vi "Custom Device CORE.vi"(8 "error in (no error)":errorcluster, 11 "CDW_MetaDataObj":refnum<class "NIVS_Consolidated_CDW_MetaDataObj.lvclass">) -> (0 "error out":errorcluster)   [LabVIEW 2015, in "NIVS_Consolidated_CDW_MetaDataObj.lvclass"]
doc: "This VI is the Core VI for the Custom Device Wizard.\n\nWritten by:\nStephan Daunke\n\nDate:\n2014/01/27\n\nCompany:\nNational Instruments Germany GmbH"
uses:
  NIVS_Consolidated_CDW_MetaDataObj.lvclass
  Action.ctl
  Internal data.ctl
  <resource>/dialog/NewProjectWizard/MetaDataObj/MetaDataObj.lvclass/MetaDataObj.ctl
  NIVS_Consolidated_CDW_MetaDataObj.lvclass/NIVS_Consolidated_CDW_MetaDataObj.ctl
  Template Classes/NIVS_CD Template/NIVS_CD Template.lvclass/NIVS_CD Template.ctl
  Utility folder.ctl
  CD Shared lvlib.ctl
  Common.ctl
  Add Item - Type.ctl
  CD System Explorer lvlib.ctl
  <vilib>/Utility/traverseref.llb/TRef TravTarget.ctl
  CD Engine lvlib.ctl
  Build Spec System Explorer.ctl
  Build Spec Engine.ctl
  <resource>/dialog/NewProjectWizard/MetaDataObj/Accessors/Read Project Root.vi
  Read CD Template.vi
  Template Classes/NIVS_CD Template/Read Extra Page Names.vi
  <resource>/dialog/NewProjectWizard/MetaDataObj/Accessors/Read Project Name.vi
  Utility folder.vi
  CD Shared lvlib.vi
  Common.vi
  CD System Explorer lvlib.vi
  CD Engine lvlib.vi
  <vilib>/Utility/config.llb/Write Key (String).vi
  <vilib>/Utility/config.llb/Write Key (Path).vi
  Build Spec System Explorer.vi
  Build Spec Engine.vi
  Template Classes/NIVS_CD Template/NIVS_CD Template.lvclass
  <vilib>/Utility/config.llb/NI_LVConfig.lvlib
  <vilib>/Utility/Data Type/NI_Data Type.lvlib
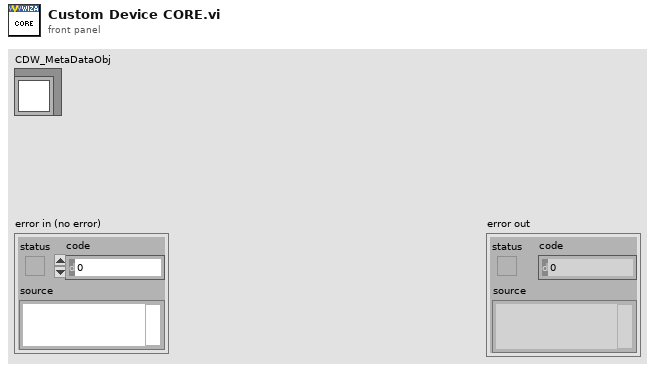
[diagram p1: front panel]
types:
  T1 = typedef "NIVS_Consolidated_CDW_MetaDataObj.lvclass/Internal data.ctl" = cluster{"CD GUID":string, "Extra Page GUIDs":string[], "System Explorer Library":refnum<vi>, "Shared Library":refnum<vi>, "Engine Library":refnum<vi>}
  T2 = typedef "NIVS_Consolidated_CDW_MetaDataObj.lvclass/Action.ctl" = enum16{"Project - Create Custom Device folder", "PC - Create GUID for each extra page", "PC-Utility - Create folder and copy -Copy .LLB to NI VeriStand dir-", "PC-Utility - Change -Copy .LLB to NI VeriStand dir-", "PC-Shared - Create folder and copy Constants.vi", "PC-Shared - Change Constants.vi content", "PC-Shared - Create library", "PC-Shared - Add folders and VIs to library", "PC-System Explorer - Create folder and copy templates", "PC-System Explorer - Create extra pages", "PC-System Explorer - Create library", "PC-System Explorer - Add folders and VIs to library", "PC-Engine - Create folder and copy the RT Template", "PC-Engine - Create library", "PC-Engine - Add virtual folders and VIs to library", "PC-XML - Create and change file", "PC-Help - Copy HTML Files", "Project - Read project file content", "Project - Edit Utility section", "Project - Edit XML section", "Project - Edit Engine Library section", "Project - Edit Shared Library section", "Project - Edit System Explorer Library section", "Project - Edit Custom Device Name", "Project - Edit System Explorer LLB Name", "Project - Edit Engine LLB OS dependent file name", "Project - Write new project file"}
  T3 = typedef "NIVS_Consolidated_CDW_MetaDataObj.lvclass/Utility folder.ctl" = enum16{"Utility.FolderName", "Utility.Copy .llb to NI VeriStand dir.FileName", "Utility.Copy .llb to NI VeriStand dir.FilePathAndName", "Utility.LLB Pre Build.FilePathAndName"}
  T4 = typedef "NIVS_Consolidated_CDW_MetaDataObj.lvclass/CD Shared lvlib.ctl" = enum16{"LibraryFileName", "LibraryFolderName", "ConstantsVI.VIPathAndName", "Shared.FolderName", "Shared.Types.FolderName", "Shared.Constants.VIName", "Shared.Constants.VITemplateName", "Shared.Constants.VITemplatePathAndName", "Shared.CompiledSettings.RelativePath", "Shared.Constants.RelativePath", "Shared.CompiledSettings.Name", "Shared.CompiledSettings.Name.NoExtension", "Shared.CompiledSettings.ClusterName"}
  T5 = typedef "NIVS_Consolidated_CDW_MetaDataObj.lvclass/Common.ctl" = enum16{"ProjectName", "TemplatesFolderName", "ProjectTemplatePathAndName", "TimingAndSyncFolderName", "CustomDeviceFolderName", "PathToTemplates"}
  T6 = typedef "NIVS_Consolidated_CDW_MetaDataObj.lvclass/Add Item - Type.ctl" = string
  T7 = typedef "NIVS_Consolidated_CDW_MetaDataObj.lvclass/CD System Explorer lvlib.ctl" = enum16{"LibraryFileName", "LibraryFolderName", "System Explorer.FolderName", "System Explorer.Dynamically Called.FolderName", "System Explorer.Dynamically Called.Extra Pages.FolderName", "System Explorer.Dynamically Called.Extra Pages.TemplatePathAndName", "System Explorer.Dynamically Called.Main Page.VIName", "System Explorer.Dynamically Called.Main Page.TemplatePathAndName", "System Explorer.Dynamically Called.Initialization VI.VIName", "System Explorer.Dynamically Called.Initialization VI.TemplatePathAndName", "System Explorer.SubVI.FolderName", "System Explorer.Types.FolderName", "System Explorer.ActionVIOnCompile.VIName", "System Explorer.ExportConfigRTM.VIName", "System Explorer.LoadHelpFile.VIName"}
  T8 = typedef "TRef TravTarget.ctl" = enum16{"FP", "BD", "Other"}
  T9 = typedef "NIVS_Consolidated_CDW_MetaDataObj.lvclass/CD Engine lvlib.ctl" = enum16{"LibraryFileName", "LibraryFolderName", "Engine.FolderName", "Engine.Init.FolderName", "Engine.Run.FolderName", "Engine.Shutdown.FolderName", "Types.FolderName", "Engine.RT Driver VI.TemplatePath", "Engine.RT Driver VI.FileName", "Engine.RTStateVariables.Name", "Engine.RTStateVariables.Name.NoExtension", "Engine.Async.NameExtension", "Engine.Async.TemplateName"}
  T10 = typedef "NIVS_Consolidated_CDW_MetaDataObj.lvclass/Build Spec System Explorer.ctl" = enum16{"Destinations.LLBFileName"}
  T11 = typedef "NIVS_Consolidated_CDW_MetaDataObj.lvclass/Build Spec Engine.ctl" = enum16{"Destinations.LLBWindowsFileName", "Destinations.LLBVxWorksFileName", "Destinations.LLBPharlapFileName", "Destinations.LLBLinuxARMFileName", "Destinations.LLBLinux64FileName"}
  T12 = enum16{"open", "replace", "create", "open or create", "replace or create", "replace or create with confirmation"}
  T13 = typedef "NI_LVConfig.lvlib/Config Data RefNum.ctl" = refnum<k1>
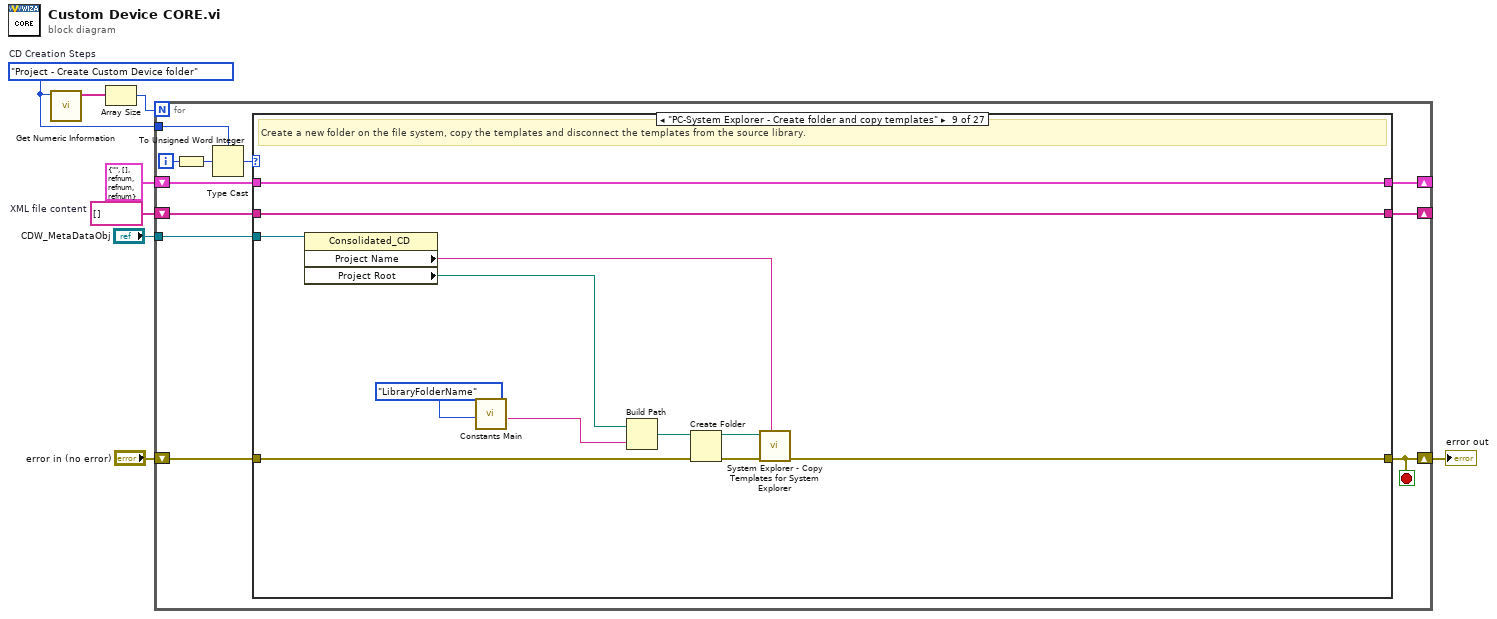
[diagram p0: block diagram]
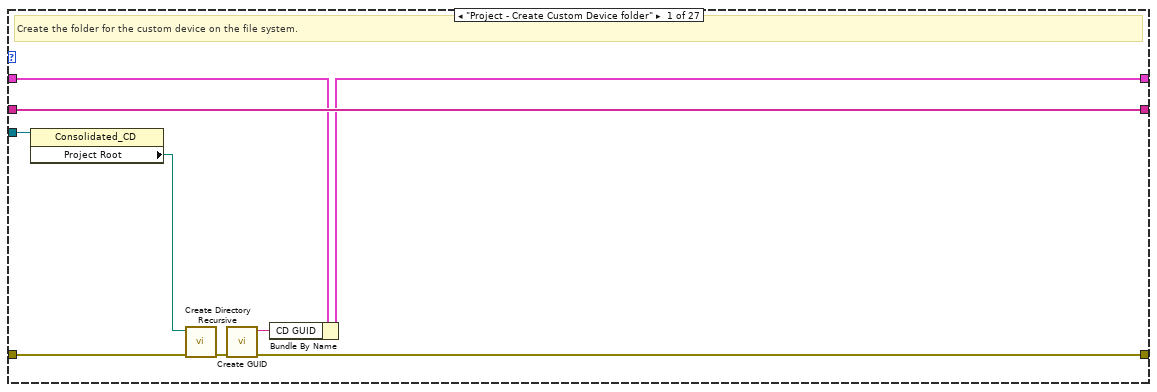
[diagram p2: hidden frame]
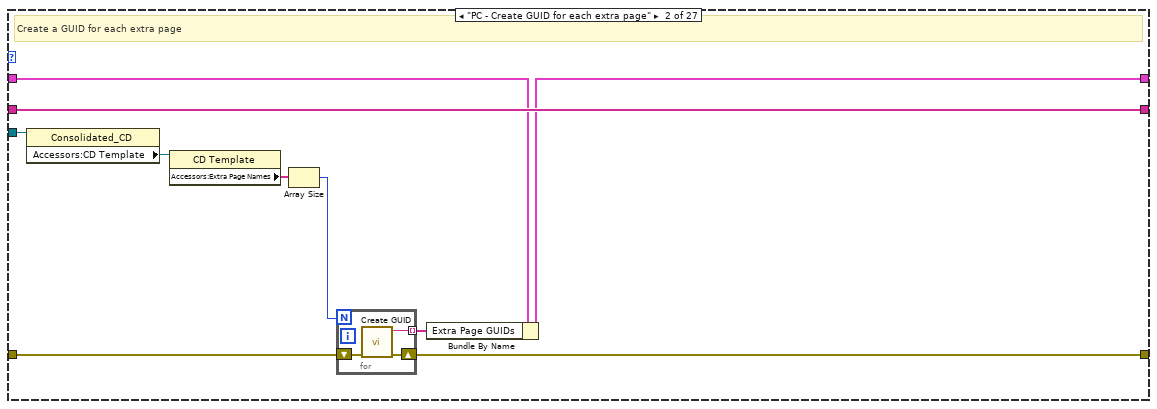
[diagram p3: hidden frame]
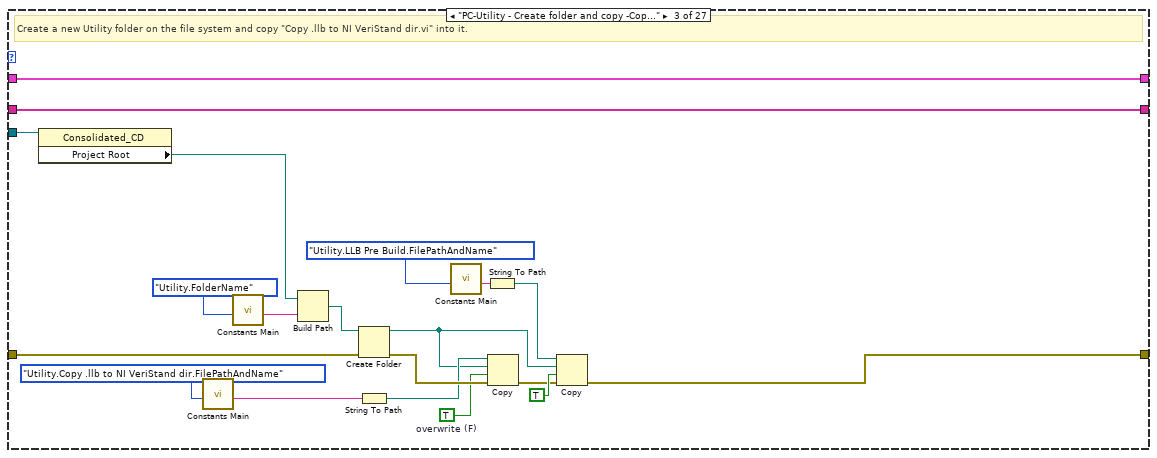
[diagram p4: hidden frame]
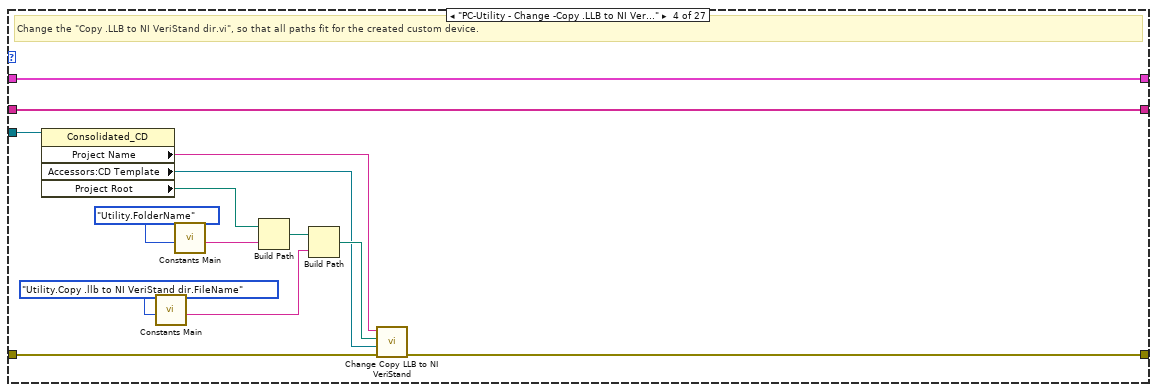
[diagram p5: hidden frame]
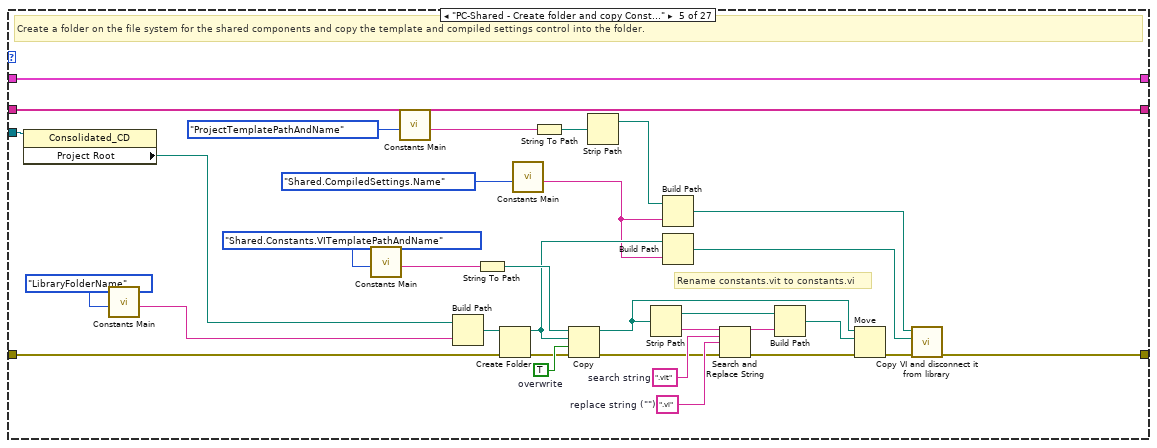
[diagram p6: hidden frame]
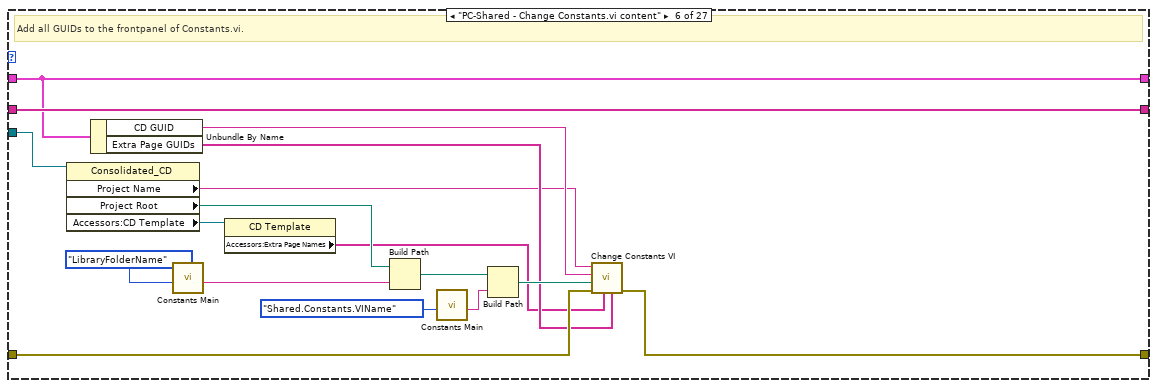
[diagram p7: hidden frame]
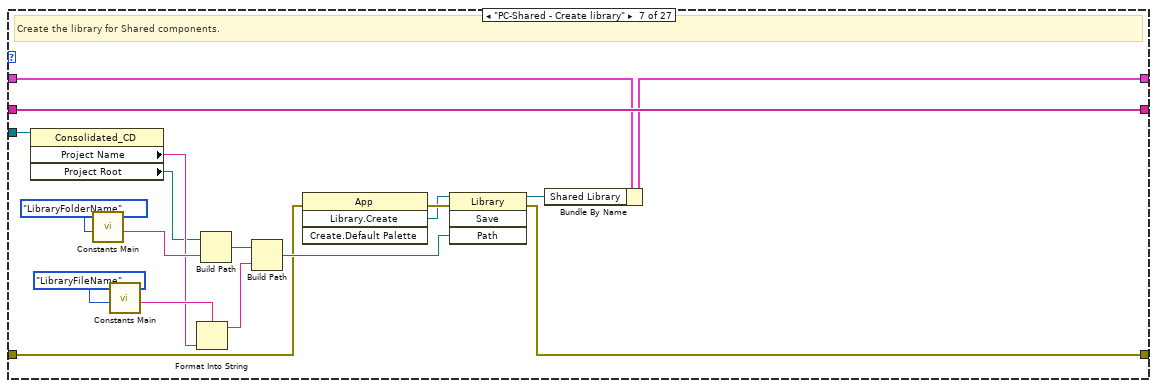
[diagram p8: hidden frame]
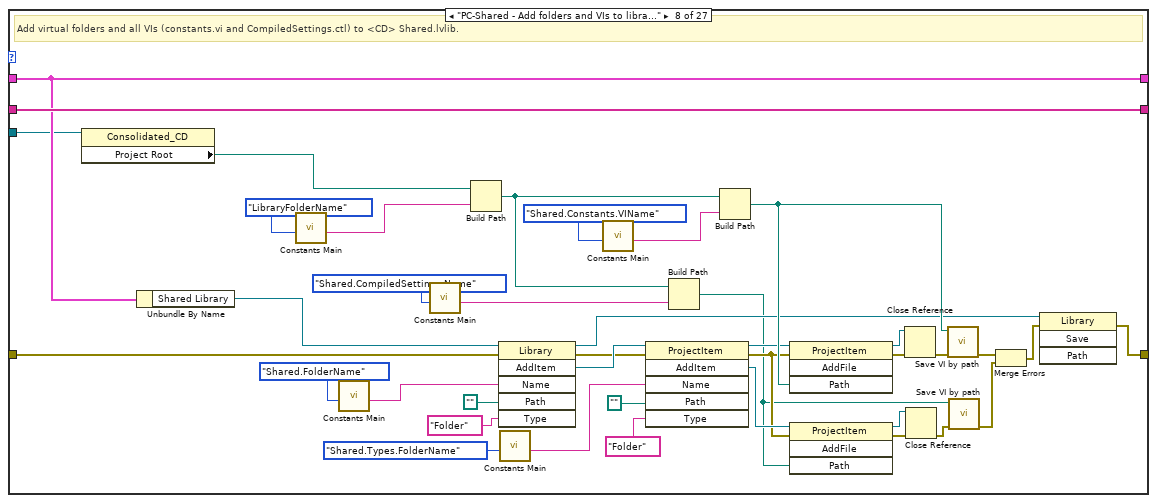
[diagram p9: hidden frame]
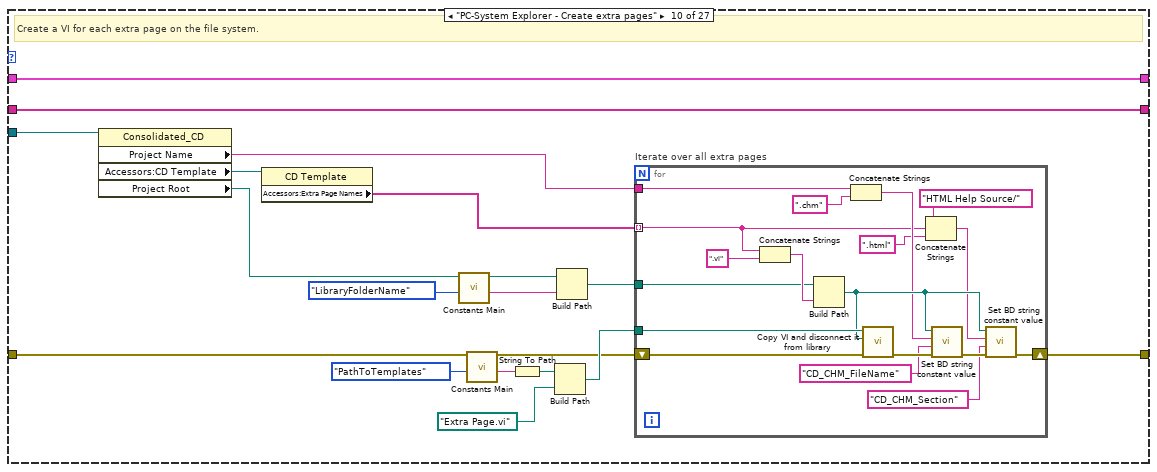
[diagram p10: hidden frame]
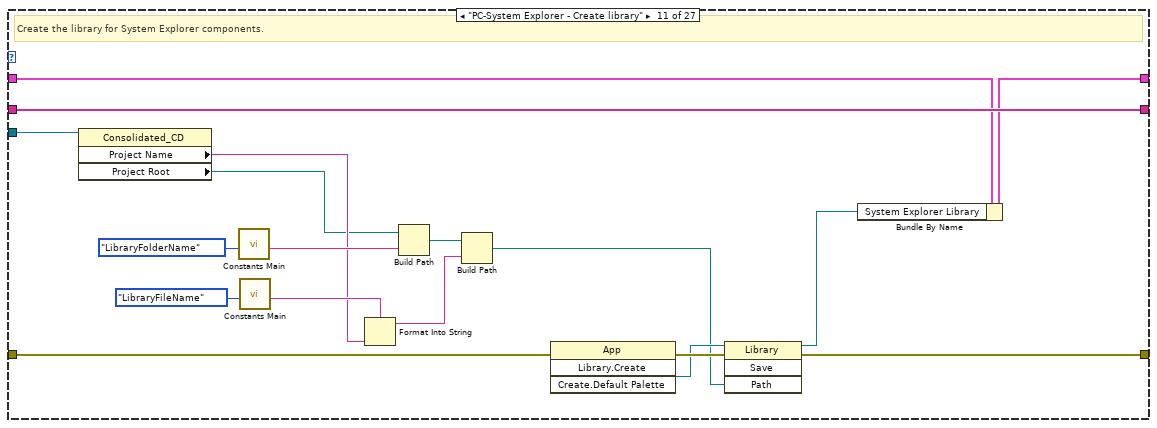
[diagram p11: hidden frame]
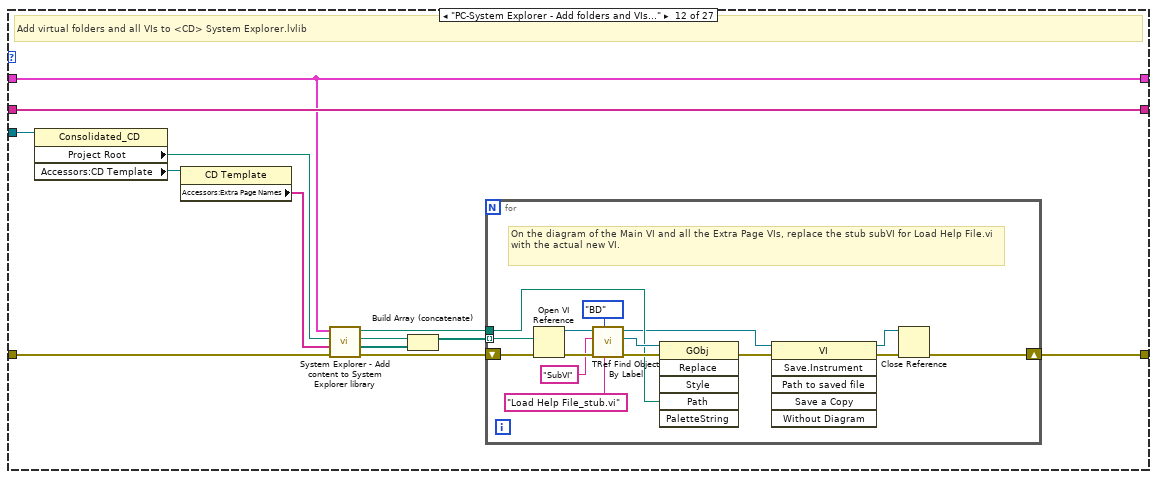
[diagram p12: hidden frame]
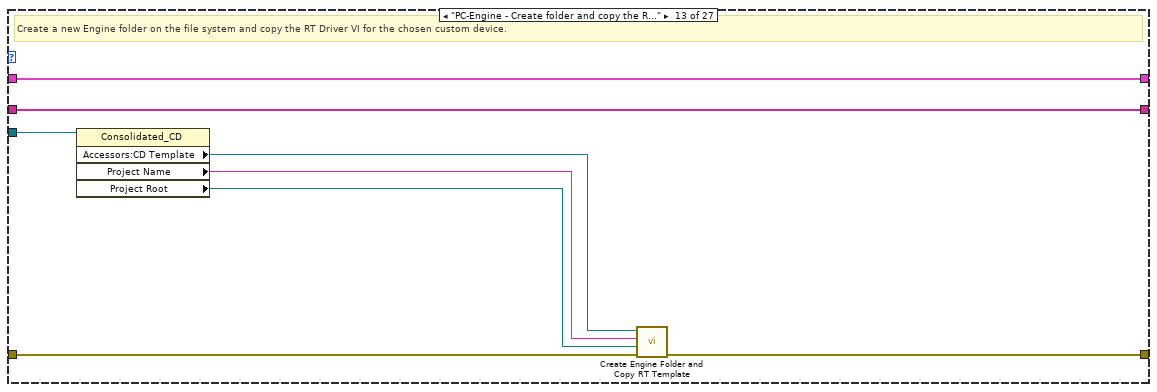
[diagram p13: hidden frame]
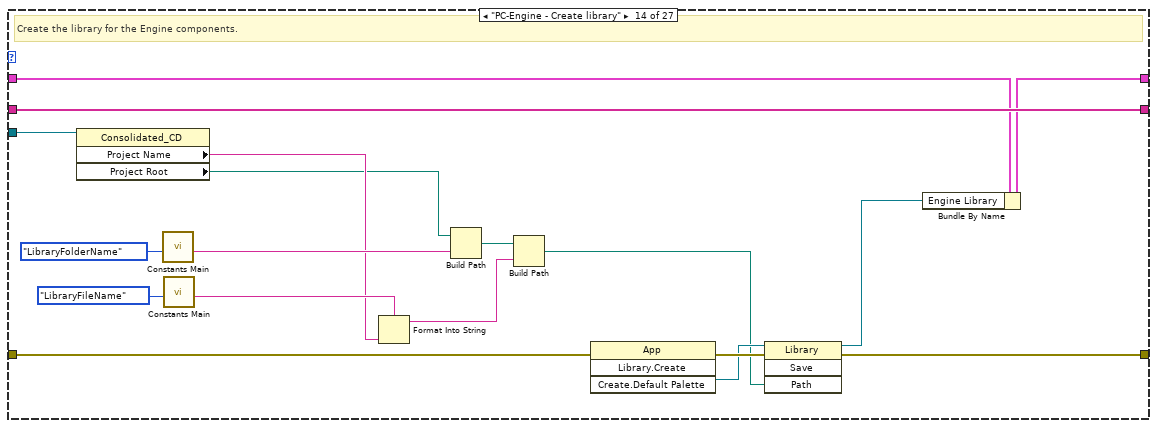
[diagram p14: hidden frame]
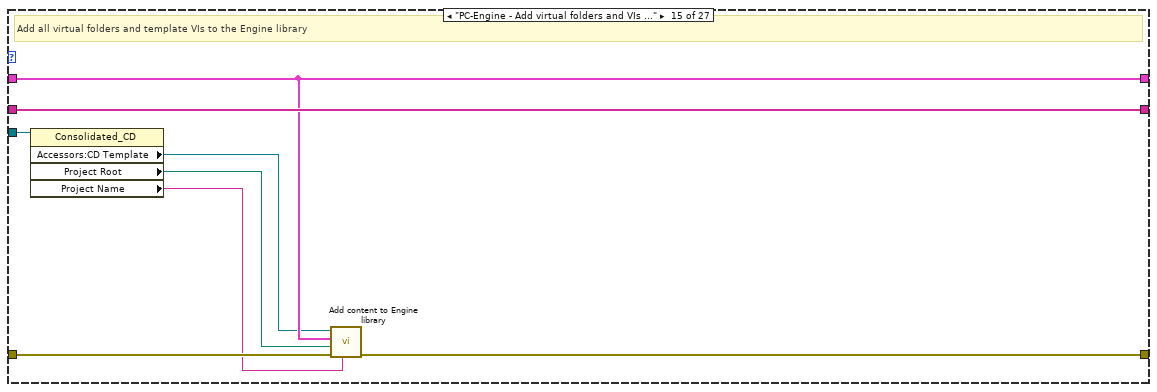
[diagram p15: hidden frame]
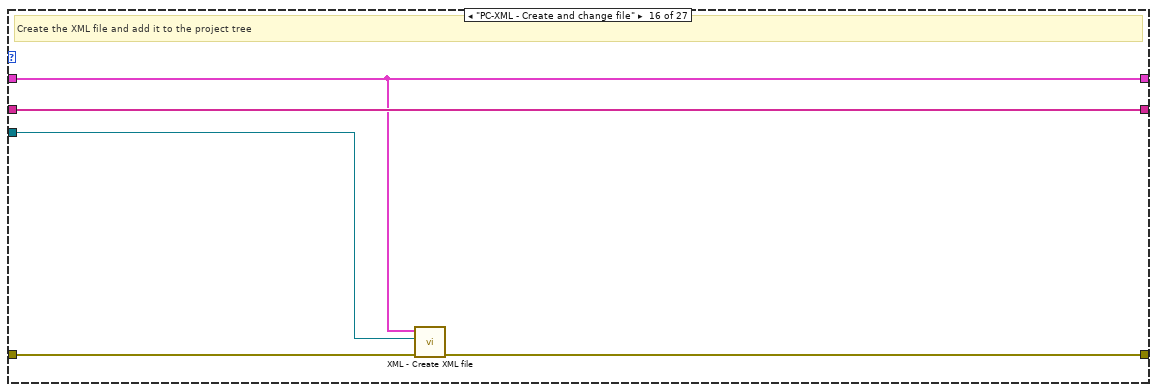
[diagram p16: hidden frame]
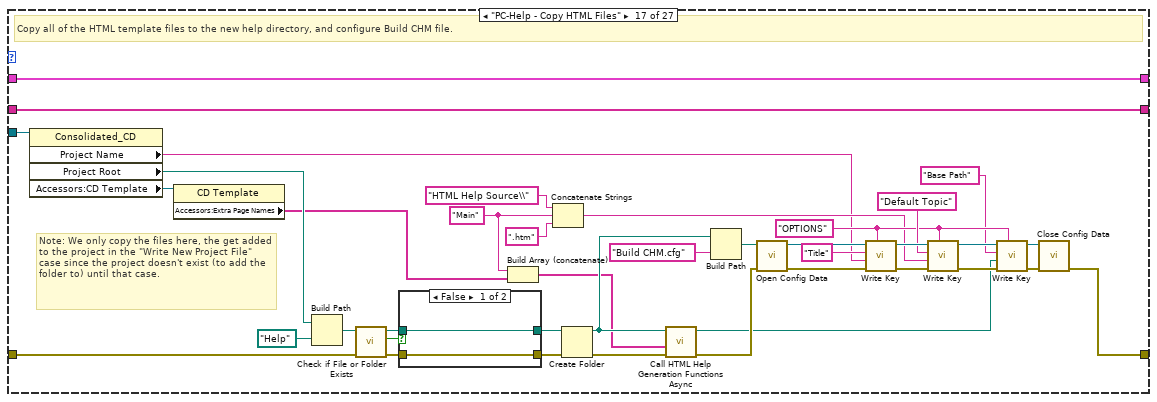
[diagram p17: hidden frame]
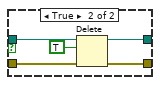
[diagram p18: hidden frame]
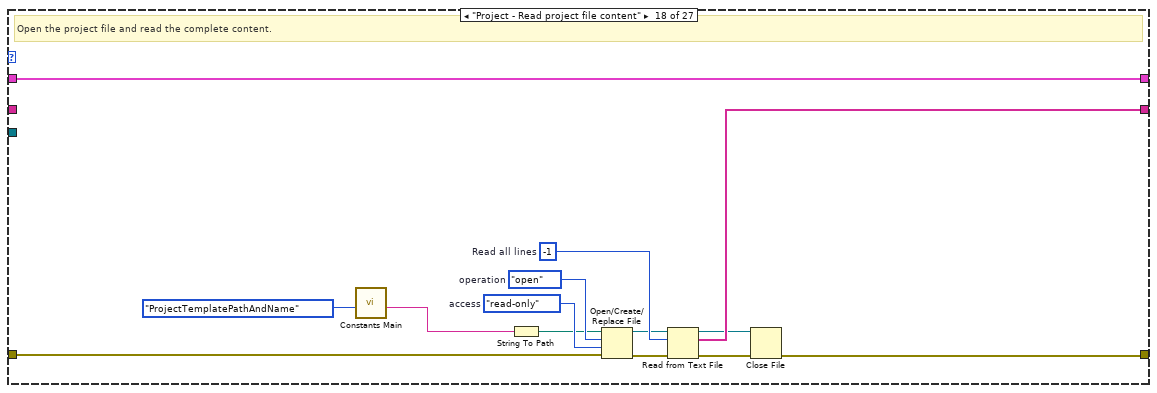
[diagram p19: hidden frame]
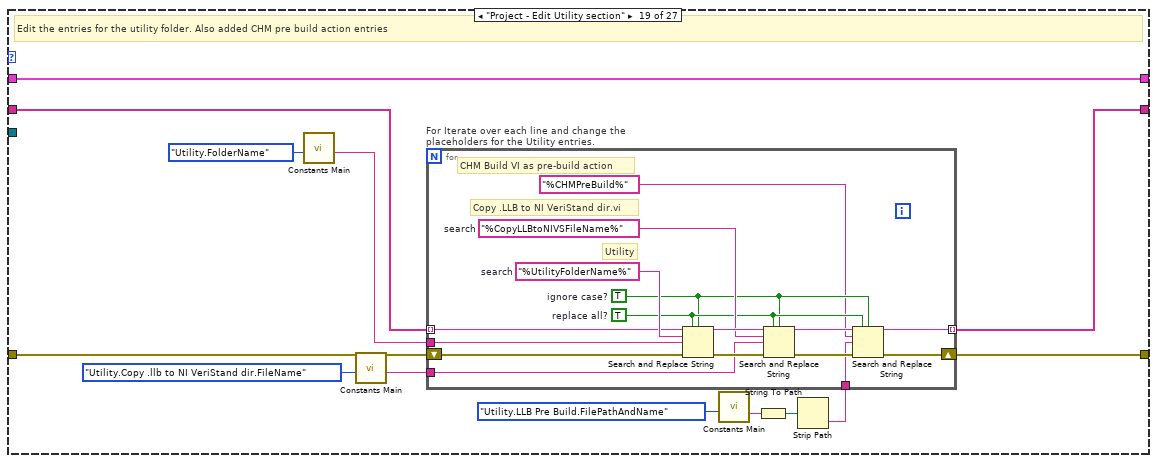
[diagram p20: hidden frame]
diagram:
  w4 = Action."Project - Create Custom Device folder"  # CD Creation Steps
  w5 = string[] []  # XML file content
  n1 = call <vilib>:"Get Numeric Information.vi"("Variant"=w4) -> ("Enum Names"=w3:string[])  [unwired: 7 in, 3 out]
  n2 = Array Size(array=w3) -> (size(s)=w2:i32)
  n3 = for {
    N: w2 -> [_]
    shift-right: [w16] -> _
    shift-left: T1 {"CD GUID"="", "Extra Page GUIDs"=[], "System Explorer Library"=refnum, "Shared Library"=refnum, "Engine Library"=refnum} ("CD Wizard - Internal Data") -> [w18]
    shift-right: [w15] -> _
    shift-left: w5 -> [w17]
    shift-right: [w14] -> w6
    shift-left: "error in (no error)" -> [w19]
    tunnel: w4 -> [w12]
    tunnel: "CDW_MetaDataObj" -> [w11]
    i -> [w13]
    stop <- w14 stop-if-true
    n4 = To Unsigned Word Integer(number=w13) -> (unsigned 16bit integer=w9:u16)
    n5 = Type Cast(type=w12, x=w9) -> (*(type *) &x=w10:T2)
    n6 = case shown="\"PC-System Explorer - Create folder and copy templates\"" w10 {
      tunnel: w19 -> [w24 w37 w43 w63 w78 w118 w129 w145 w183 w200 w233 w259 w282 w287 w308 w313 w331 w361 w374 w406 w425 w429 w459 w493 w504 w522 w560]
      tunnel: [w25 w36 w47 w69 w80 w124 w130 w163 w188 w210 w234 w254 w281 w290 w307 w312 w330 w367 w383 w411 w424 w439 w463 w492 w511 w534 w567] -> w14
      tunnel: w18 -> [w22 w34 w46 w67 w79 w115 w133 w164 w187 w209 w239 w257 w280 w294 w305 w311 w326 w373 w386 w408 w423 w430 w460 w489 w508 w540 w592]
      tunnel: w17 -> [w28 w38 w61 w75 w108 w125 w143 w182 w194 w211 w247 w260 w283 w301 w309 w314 w353 _ w385 w410 w422 w434 w461 w490 w506 w535 w586]
      tunnel: [w27 w33 w46 w67 w79 w115 w132 w164 w187 w209 w240 w257 w280 w293 w305 w311 w326 w373 w386 w408 w423 w430 w460 w489 w508 w540 w592] -> w16
      tunnel: [w28 w38 w61 w75 w108 w125 w143 w182 w194 w211 w247 w260 w283 w301 w309 w314 w353 w366 w384 w409 w426 w440 w462 w491 w505 w523 w586] -> w15
      tunnel: w11 -> [w21 w32 w45 w66 w77 w117 w128 w147 w186 w199 w232 w253 w279 w286 w306 w310 w319 _ _ w405 w421 w428 w458 w488 w503 w521 w559]
      frame "Project - Create Custom Device folder" {
        # "Create the folder for the custom device on the file system."
        n7 = property class="Consolidated_CD"(reference=w21) -> ("Project Root"=w20:path)  [unwired: 1 in, 2 out]
        n8 = call <vilib>:"Create Directory Recursive.vi"("error in (no error)"=w24, "directory"=w20) -> ("error out"=w23:errorcluster)  [unwired: 3 in, 2 out]
        n9 = call "Create GUID.vi"("error in (no error)"=w23) -> ("error out"=w25:errorcluster, "Generated GUID"=w26:string)  [unwired: 9 in]
        n10 = Bundle By Name(cluster=w22, "CD GUID"=w26) -> (w27:T1)
      }
      frame "PC - Create GUID for each extra page" {
        # "Create a GUID for each extra page"
        n11 = property class="Consolidated_CD"(reference=w32) -> ("Accessors:CD Template"=w31:refnum<class "NIVS_CD Template.lvclass">)  [unwired: 1 in, 2 out]
        n12 = property class="CD Template"(reference=w31) -> ("Accessors:Extra Page Names"=w30:string[])  [unwired: 1 in, 2 out]
        n13 = Array Size(array=w30) -> (size(s)=w29:i32)
        n14 = for {
          N: w29 -> [_]
          shift-right: [w40] -> w36
          shift-left: w37 -> [w41]
          tunnel: [w39] -> w35 mode=indexing
          n15 = call "Create GUID.vi"("error in (no error)"=w41) -> ("error out"=w40:errorcluster, "Generated GUID"=w39:string)  [unwired: 9 in]
        }
        n16 = Bundle By Name(cluster=w34, "Extra Page GUIDs"=w35) -> (w33:T1)
      }
      frame "PC-Utility - Create folder and copy -Copy .LLB to NI VeriStand dir-" {
        w58 = TRUE  # overwrite (F)
        # "Create a new Utility folder on the file system and copy \"Copy .llb to NI VeriStand dir.vi\" into it."
        n17 = property class="Consolidated_CD"(reference=w45) -> ("Project Root"=w44:path)  [unwired: 1 in, 2 out]
        n18 = call-poly "Constants Main.vi"("Action"=Utility_folder."Utility.Copy .llb to NI VeriStand dir.FilePathAndName") -> ("Output"=w56:string)  [unwired: 10 in]
        n19 = call-poly "Constants Main.vi"("Action"=Utility_folder."Utility.FolderName") -> ("Output"=w53:string)  [unwired: 10 in]
        n20 = Build Path(base path=w44, name or relative path=w53) -> (appended path=w60:path)
        n21 = Create Folder(path (use dialog)=w60, error in=w43) -> (created path=w52:path, error out=w59:errorcluster)  [unwired: 1 in, 1 out]
        n22 = String To Path(string=w56) -> (path=w55:path)
        n23 = call-poly "Constants Main.vi"("Action"=Utility_folder."Utility.LLB Pre Build.FilePathAndName") -> ("Output"=w50:string)  [unwired: 10 in]
        n24 = String To Path(string=w50) -> (path=w49:path)
        n25 = Copy(8:w59, 9:w58, 10:w52, 11:w55) -> (0:w42:errorcluster)  [unwired: 3 out]
        n26 = Copy(8:w42, 9:TRUE ("overwrite (F)"), 10:w52, 11:w49) -> (0:w47:errorcluster)  [unwired: 3 out]
      }
      frame "PC-Utility - Change -Copy .LLB to NI VeriStand dir-" {
        # "Change the \"Copy .LLB to NI VeriStand dir.vi\", so that all paths fit for the created custom device."
        n27 = property class="Consolidated_CD"(reference=w66) -> ("Project Name"=w65:string, "Accessors:CD Template"=w64:refnum<class "NIVS_CD Template.lvclass">, "Project Root"=w62:path)  [unwired: 1 in, 2 out]
        n28 = call-poly "Constants Main.vi"("Action"=Utility_folder."Utility.Copy .llb to NI VeriStand dir.FileName") -> ("Output"=w70:string)  [unwired: 10 in]
        n29 = call-poly "Constants Main.vi"("Action"=Utility_folder."Utility.FolderName") -> ("Output"=w72:string)  [unwired: 10 in]
        n30 = Build Path(base path=w62, name or relative path=w72) -> (appended path=w71:path)
        n31 = Build Path(base path=w71, name or relative path=w70) -> (appended path=w68:path)
        n32 = call "Change Copy LLB to NI VeriStand.vi"("error in (no error)"=w63, "CD Template"=w64, "Copy .LLB to ... path"=w68, "CD Name"=w65) -> ("error out"=w69:errorcluster)  [unwired: 7 in]
      }
      frame "PC-Shared - Create folder and copy Constants.vi" {
        w97 = ".vi"  # replace string ("")
        w98 = ".vit"  # search string
        w102 = TRUE  # overwrite
        # "Rename constants.vit to constants.vi"
        # "Create a folder on the file system for the shared components and copy the template and compiled settings control into the folder."
        n33 = property class="Consolidated_CD"(reference=w77) -> ("Project Root"=w76:path)  [unwired: 1 in, 2 out]
        n34 = call-poly "Constants Main.vi"("Action"=CD_Shared_lvlib."LibraryFolderName") -> ("Output"=w105:string)  [unwired: 10 in]
        n35 = call-poly "Constants Main.vi"("Action"=CD_Shared_lvlib."Shared.Constants.VITemplatePathAndName") -> ("Output"=w103:string)  [unwired: 10 in]
        n36 = call-poly "Constants Main.vi"("Action"=Common."ProjectTemplatePathAndName") -> ("Output"=w89:string)  [unwired: 10 in]
        n37 = Build Path(base path=w76, name or relative path=w105) -> (appended path=w107:path)
        n38 = String To Path(string=w103) -> (path=w95:path)
        n39 = Create Folder(path (use dialog)=w107, error in=w78) -> (created path=w86:path, error out=w96:errorcluster)  [unwired: 1 in, 1 out]
        n40 = call-poly "Constants Main.vi"("Action"=CD_Shared_lvlib."Shared.CompiledSettings.Name") -> ("Output"=w81:string)  [unwired: 10 in]
        n41 = String To Path(string=w89) -> (path=w88:path)
        n42 = Copy(8:w96, 9:w102, 10:w86, 11:w95) -> (0:w94:errorcluster, 3:w91:path)  [unwired: 2 out]
        n43 = Strip Path(path=w88) -> (stripped path=w87:path)  [unwired: 1 out]
        n44 = Strip Path(path=w91) -> (stripped path=w101:path, name=w100:string)
        n45 = Build Path(base path=w87, name or relative path=w81) -> (appended path=w85:path)
        n46 = Build Path(base path=w86, name or relative path=w81) -> (appended path=w84:path)
        n47 = Search and Replace String(input string=w100, search string=w98, replace string=w97, error in=w94) -> (result string=w99:string, error out=w93:errorcluster)  [unwired: 4 in, 2 out]
        n48 = Build Path(base path=w101, name or relative path=w99) -> (appended path=w92:path)
        n49 = Move(source path=w91, error in=w93, 10:w92) -> (error out=w83:errorcluster)  [unwired: 2 in, 2 out]
        n50 = call "Copy VI and disconnect it from library.vi"("error in (no error)"=w83, "VI Target Path"=w84, "VI Source Path"=w85) -> ("error out"=w80:errorcluster)  [unwired: 8 in]
      }
      frame "PC-Shared - Change Constants.vi content" {
        # "Add all GUIDs to the frontpanel of Constants.vi."
        n51 = property class="Consolidated_CD"(reference=w117) -> ("Project Name"=w111:string, "Project Root"=w116:path, "Accessors:CD Template"=w110:refnum<class "NIVS_CD Template.lvclass">)  [unwired: 1 in, 2 out]
        n52 = Unbundle By Name(w115) -> ("CD GUID"=w113:string, "Extra Page GUIDs"=w112:string[])
        n53 = call-poly "Constants Main.vi"("Action"=CD_Shared_lvlib."LibraryFolderName") -> ("Output"=w119:string)  [unwired: 10 in]
        n54 = property class="CD Template"(reference=w110) -> ("Accessors:Extra Page Names"=w109:string[])  [unwired: 1 in, 2 out]
        n55 = Build Path(base path=w116, name or relative path=w119) -> (appended path=w123:path)
        n56 = call-poly "Constants Main.vi"("Action"=CD_Shared_lvlib."Shared.Constants.VIName") -> ("Output"=w121:string)  [unwired: 10 in]
        n57 = Build Path(base path=w123, name or relative path=w121) -> (appended path=w114:path)
        n58 = call "Change Constants VI.vi"("Extra Page GUIDs"=w112, "Extra Page Names"=w109, "error in (no error)"=w118, "Constants.vi path"=w114, "CD GUID"=w113, "CD Name"=w111) -> ("error out"=w124:errorcluster)  [unwired: 5 in]
      }
      frame "PC-Shared - Create library" {
        # "Create the library for Shared components."
        n59 = property class="Consolidated_CD"(reference=w128) -> ("Project Name"=w127:string, "Project Root"=w126:path)  [unwired: 1 in, 2 out]
        n60 = call-poly "Constants Main.vi"("Action"=CD_Shared_lvlib."LibraryFolderName") -> ("Output"=w137:string)  [unwired: 10 in]
        n61 = call-poly "Constants Main.vi"("Action"=CD_Shared_lvlib."LibraryFileName") -> ("Output"=w138:string)  [unwired: 10 in]
        n62 = Format Into String(format string=w138, w127) -> (resulting string=w141:string)  [unwired: 2 in, 1 out]
        n63 = Build Path(base path=w126, name or relative path=w137) -> (appended path=w142:path)
        n64 = Build Path(base path=w142, name or relative path=w141) -> (appended path=w134:path)
        n65 = invoke class="App" method="Library.Create"(error in=w129) -> (error out=w136:errorcluster, "Create Library"=w135:refnum<vi>)  [unwired: 3 in, 2 out]
        n66 = invoke class="Library" method="Save"(reference=w135, error in=w136, "Path"=w134) -> (reference out=w131:refnum<vi>, error out=w130:errorcluster)  [unwired: 1 in, 2 out]
        n67 = Bundle By Name(cluster=w133, "Shared Library"=w131) -> (w132:T1)
      }
      frame "PC-Shared - Add folders and VIs to library" {
        # "Add virtual folders and all VIs (constants.vi and CompiledSettings.ctl) to <CD> Shared.lvlib."
        n68 = property class="Consolidated_CD"(reference=w147) -> ("Project Root"=w146:path)  [unwired: 1 in, 2 out]
        n69 = Unbundle By Name(w164) -> ("Shared Library"=w166:refnum<vi>)
        n70 = call-poly "Constants Main.vi"("Action"=CD_Shared_lvlib."LibraryFolderName") -> ("Output"=w160:string)  [unwired: 10 in]
        n71 = call-poly "Constants Main.vi"("Action"=CD_Shared_lvlib."Shared.FolderName") -> ("Output"=w161:string)  [unwired: 10 in]
        n72 = call-poly "Constants Main.vi"("Action"=CD_Shared_lvlib."Shared.CompiledSettings.Name") -> ("Output"=w152:string)  [unwired: 10 in]
        n73 = Build Path(base path=w146, name or relative path=w160) -> (appended path=w157:path)
        n74 = invoke class="Library" method="AddItem"(reference=w166, error in=w145, "Name"=w161, "Path"=path "", "Type"=T6 "Folder" ("Add Item - Type")) -> (reference out=w172:refnum<vi>, error out=w167:errorcluster, "AddItem"=w169:refnum<vi>)  [unwired: 1 in, 3 out]
        n75 = call-poly "Constants Main.vi"("Action"=CD_Shared_lvlib."Shared.Types.FolderName") -> ("Output"=w180:string)  [unwired: 10 in]
        n76 = call-poly "Constants Main.vi"("Action"=CD_Shared_lvlib."Shared.Constants.VIName") -> ("Output"=w148:string)  [unwired: 10 in]
        n77 = invoke class="ProjectItem" method="AddItem"(reference=w169, error in=w167, "Name"=w180, "Path"=path "", "Type"=T6 "Folder" ("Add Item - Type")) -> (reference out=w171:refnum<vi>, error out=w158:errorcluster, "AddItem"=w159:refnum<vi>)  [unwired: 1 in, 3 out]
        n78 = Build Path(base path=w157, name or relative path=w152) -> (appended path=w156:path)
        n79 = Build Path(base path=w157, name or relative path=w148) -> (appended path=w173:path)
        n80 = invoke class="ProjectItem" method="AddFile"(reference=w171, error in=w158, "Path"=w173) -> (reference out=w176:refnum<vi>, error out=w175:errorcluster)  [unwired: 1 in, 2 out]
        n81 = invoke class="ProjectItem" method="AddFile"(reference=w159, error in=w158, "Path"=w156) -> (reference out=w150:refnum<vi>, error out=w149:errorcluster)  [unwired: 1 in, 2 out]
        n82 = Close Reference(reference=w176, error in (no error)=w175) -> (error out=w177:errorcluster)
        n83 = Close Reference(reference=w150, error in (no error)=w149) -> (error out=w151:errorcluster)
        n84 = call "Save VI by path.vi"("error in (no error)"=w177, "VI path"=w173) -> ("error out"=w174:errorcluster)  [unwired: 9 in]
        n85 = call "Save VI by path.vi"("error in (no error)"=w151, "VI path"=w156) -> ("error out"=w154:errorcluster)  [unwired: 9 in]
        n86 = Merge Errors(w174, w154) -> (w155:errorcluster)
        n87 = invoke class="Library" method="Save"(reference=w172, error in=w155) -> (error out=w163:errorcluster)  [unwired: 2 in, 3 out]
      }
      frame "PC-System Explorer - Create folder and copy templates" {
        # "Create a new folder on the file system, copy the templates and disconnect the templates from the source library."
        n88 = property class="Consolidated_CD"(reference=w186) -> ("Project Name"=w185:string, "Project Root"=w184:path)  [unwired: 1 in, 2 out]
        n89 = call-poly "Constants Main.vi"("Action"=CD_System_Explorer_lvlib."LibraryFolderName") -> ("Output"=w191:string)  [unwired: 10 in]
        n90 = Build Path(base path=w184, name or relative path=w191) -> (appended path=w193:path)
        n91 = Create Folder(path (use dialog)=w193, error in=w183) -> (created path=w189:path, error out=w190:errorcluster)  [unwired: 1 in, 1 out]
        n92 = call "System Explorer - Copy Templates for System Explorer.vi"("CD Name"=w185, "error in (no error)"=w190, "System Explorer folder"=w189) -> ("error out"=w188:errorcluster)  [unwired: 8 in]
      }
      frame "PC-System Explorer - Create extra pages" {
        # "Create a VI for each extra page on the file system."
        n93 = property class="Consolidated_CD"(reference=w199) -> ("Project Name"=w198:string, "Accessors:CD Template"=w197:refnum<class "NIVS_CD Template.lvclass">, "Project Root"=w195:path)  [unwired: 1 in, 2 out]
        n94 = property class="CD Template"(reference=w197) -> ("Accessors:Extra Page Names"=w196:string[])  [unwired: 1 in, 2 out]
        n95 = call-poly "Constants Main.vi"("Action"=CD_System_Explorer_lvlib."LibraryFolderName") -> ("Output"=w207:string)  [unwired: 10 in]
        n96 = call-poly "Constants Main.vi"("Action"=Common."PathToTemplates") -> ("Output"=w203:string)  [unwired: 10 in]
        n97 = String To Path(string=w203) -> (path=w202:path)
        n98 = Build Path(base path=w202, name or relative path=path "Extra Page.vi") -> (appended path=w208:path)
        n99 = Build Path(base path=w195, name or relative path=w207) -> (appended path=w205:path)
        n100 = for "Iterate over all extra pages" {
          tunnel: w196 -> [w213] mode=indexing
          shift-right: [w218] -> w210
          shift-left: w200 -> [w227]
          tunnel: w205 -> [w225]
          tunnel: w208 -> [w226]
          tunnel: w198 -> [w222]
          n101 = Concatenate Strings(w213, ".vi") -> (w228:string)
          n102 = Build Path(base path=w225, name or relative path=w228) -> (appended path=w220:path)
          n103 = Concatenate Strings(w222, ".chm" ("string")) -> (w217:string)
          n104 = call "Copy VI and disconnect it from library.vi"("error in (no error)"=w227, "VI Target Path"=w220, "VI Source Path"=w226) -> ("error out"=w224:errorcluster)  [unwired: 8 in]
          n105 = Concatenate Strings("HTML Help Source/" ("string"), w213, ".html" ("string")) -> (w215:string)
          n106 = call "Set BD string constant value.vi"("error in (no error)"=w224, "Name of string constant"="CD_CHM_FileName", "New String Value"=w217, "Path to VI"=w220) -> ("error out"=w221:errorcluster)  [unwired: 7 in]
          n107 = call "Set BD string constant value.vi"("error in (no error)"=w221, "Name of string constant"="CD_CHM_Section", "New String Value"=w215, "Path to VI"=w220) -> ("error out"=w218:errorcluster)  [unwired: 7 in]
        }
      }
      frame "PC-System Explorer - Create library" {
        # "Create the library for System Explorer components."
        n108 = property class="Consolidated_CD"(reference=w232) -> ("Project Name"=w231:string, "Project Root"=w230:path)  [unwired: 1 in, 2 out]
        n109 = call-poly "Constants Main.vi"("Action"=CD_System_Explorer_lvlib."LibraryFolderName") -> ("Output"=w243:string)  [unwired: 10 in]
        n110 = call-poly "Constants Main.vi"("Action"=CD_System_Explorer_lvlib."LibraryFileName") -> ("Output"=w244:string)  [unwired: 10 in]
        n111 = Format Into String(format string=w244, w231) -> (resulting string=w245:string)  [unwired: 2 in, 1 out]
        n112 = Build Path(base path=w230, name or relative path=w243) -> (appended path=w246:path)
        n113 = Build Path(base path=w246, name or relative path=w245) -> (appended path=w235:path)
        n114 = invoke class="App" method="Library.Create"(error in=w233) -> (error out=w238:errorcluster, "Create Library"=w237:refnum<vi>)  [unwired: 3 in, 2 out]
        n115 = invoke class="Library" method="Save"(reference=w237, error in=w238, "Path"=w235) -> (reference out=w236:refnum<vi>, error out=w234:errorcluster)  [unwired: 1 in, 2 out]
        n116 = Bundle By Name(cluster=w239, "System Explorer Library"=w236) -> (w240:T1)
      }
      frame "PC-System Explorer - Add folders and VIs to library" {
        # "Add virtual folders and all VIs to <CD> System Explorer.lvlib"
        n117 = property class="Consolidated_CD"(reference=w253) -> ("Project Root"=w252:path, "Accessors:CD Template"=w251:refnum<class "NIVS_CD Template.lvclass">)  [unwired: 1 in, 2 out]
        n118 = property class="CD Template"(reference=w251) -> ("Accessors:Extra Page Names"=w250:string[])  [unwired: 1 in, 2 out]
        n119 = call "System Explorer - Add content to System Explorer library.vi"("error in (no error)"=w259, "Extra Page Names"=w250, "Project Root"=w252, "CD Wizard - Internal Data"=w257) -> ("error out"=w258:errorcluster, "Extra Page VIs"=w248:path[], "System Explorer Main VI"=w256:path, "Load Help File VI"=w255:path)  [unwired: 4 in]
        n120 = Build Array (concatenate)(w256, w248) -> (w249:path[])
        n121 = for {
          tunnel: w249 -> [w266] mode=indexing
          tunnel: w255 -> [w265]
          shift-right: [w262] -> w254
          shift-left: w258 -> [w275]
          # "On the diagram of the Main VI and all the Extra Page VIs, replace the stub subVI for Load Help File.vi with the actual new VI."
          n122 = Open VI Reference(vi path=w266, error in (no error)=w275) -> (vi reference=w272:refnum<vi>, error out=w274:errorcluster)  [unwired: 4 in]
          n123 = call <vilib>:"TRef Find Object By Label.vi"("Label"="Load Help File_stub.vi", "Traverse Target"=TRef_TravTarget."BD", "error in (no error)"=w274, "Class Name"="SubVI", "VI Ref"=w272) -> ("error out"=w273:errorcluster, "Found Obj Ref"=w267:refnum<vi>, "dup VI Ref"=w263:refnum<vi>)  [unwired: 3 in, 1 out]
          n124 = invoke class="GObj" method="Replace"(reference=w267, error in=w273, "Path"=w265) -> (error out=w268:errorcluster)  [unwired: 3 in, 5 out]
          n125 = invoke class="VI" method="Save.Instrument"(reference=w263, error in=w268) -> (reference out=w261:refnum<vi>, error out=w264:errorcluster)  [unwired: 4 in, 4 out]
          n126 = Close Reference(reference=w261, error in (no error)=w264) -> (error out=w262:errorcluster)
        }
      }
      frame "PC-Engine - Create folder and copy the RT Template" {
        # "Create a new Engine folder on the file system and copy the RT Driver VI for the chosen custom device."
        n127 = property class="Consolidated_CD"(reference=w279) -> ("Accessors:CD Template"=w276:refnum<class "NIVS_CD Template.lvclass">, "Project Name"=w278:string, "Project Root"=w277:path)  [unwired: 1 in, 2 out]
        n128 = call-dynamic "Create Engine Folder and Copy RT Template.vi"("error in (no error)"=w282, "Project Root"=w277, "Project Name"=w278, "CD Template"=w276) -> ("error out"=w281:errorcluster)  [unwired: 7 in]
      }
      frame "PC-Engine - Create library" {
        # "Create the library for the Engine components."
        n129 = property class="Consolidated_CD"(reference=w286) -> ("Project Name"=w285:string, "Project Root"=w284:path)  [unwired: 1 in, 2 out]
        n130 = call-poly "Constants Main.vi"("Action"=CD_Engine_lvlib."LibraryFolderName") -> ("Output"=w297:string)  [unwired: 10 in]
        n131 = call-poly "Constants Main.vi"("Action"=CD_Engine_lvlib."LibraryFileName") -> ("Output"=w298:string)  [unwired: 10 in]
        n132 = Format Into String(format string=w298, w285) -> (resulting string=w299:string)  [unwired: 2 in, 1 out]
        n133 = Build Path(base path=w284, name or relative path=w297) -> (appended path=w300:path)
        n134 = Build Path(base path=w300, name or relative path=w299) -> (appended path=w288:path)
        n135 = invoke class="App" method="Library.Create"(error in=w287) -> (error out=w292:errorcluster, "Create Library"=w291:refnum<vi>)  [unwired: 3 in, 2 out]
        n136 = invoke class="Library" method="Save"(reference=w291, error in=w292, "Path"=w288) -> (reference out=w289:refnum<vi>, error out=w290:errorcluster)  [unwired: 1 in, 2 out]
        n137 = Bundle By Name(cluster=w294, "Engine Library"=w289) -> (w293:T1)
      }
      frame "PC-Engine - Add virtual folders and VIs to library" {
        # "Add all virtual folders and template VIs to the Engine library"
        n138 = property class="Consolidated_CD"(reference=w306) -> ("Accessors:CD Template"=w304:refnum<class "NIVS_CD Template.lvclass">, "Project Root"=w303:path, "Project Name"=w302:string)  [unwired: 1 in, 2 out]
        n139 = call-dynamic "Add content to Engine library.vi"("Project Name"=w302, "error in (no error)"=w308, "Project Root"=w303, "CD Wizard - Internal Data"=w305, "CD Template"=w304) -> ("error out"=w307:errorcluster)  [unwired: 6 in]
      }
      frame "PC-XML - Create and change file" {
        # "Create the XML file and add it to the project tree"
        n140 = call "XML - Create XML file.vi"("error in (no error)"=w313, "Consolidated_CD"=w310, "CD Wizard - Internal Data"=w311) -> ("error out"=w312:errorcluster)  [unwired: 8 in]
      }
      frame "PC-Help - Copy HTML Files" {
        w329 = "Main"
        w344 = "OPTIONS" ("section")
        # "Note: We only copy the files here, the get added to the project in the \"Write New Project File\" case since the project doesn't exist (to add the folder to) until that case."
        # "Copy all of the HTML template files to the new help directory, and configure Build CHM file."
        n141 = property class="Consolidated_CD"(reference=w319) -> ("Project Name"=w318:string, "Project Root"=w317:path, "Accessors:CD Template"=w316:refnum<class "NIVS_CD Template.lvclass">)  [unwired: 1 in, 2 out]
        n142 = property class="CD Template"(reference=w316) -> ("Accessors:Extra Page Names"=w315:string[])  [unwired: 1 in, 2 out]
        n143 = Build Path(base path=w317, name or relative path=path "Help") -> (appended path=w328:path)
        n144 = call <vilib>:"Check if File or Folder Exists.vi"("error in (no error)"=w331, "path"=w328) -> ("error out"=w337:errorcluster, "file or folder exists?"=w351:bool, "dup path"=w352:path)  [unwired: 7 in]
        n145 = case shown="False" w351 {
          tunnel: w352 -> [w355 w359]
          tunnel: [w355 w358] -> w323
          tunnel: [w354 w357] -> w338
          tunnel: w337 -> [w354 w356]
          frame False {
          }
          frame True {
            n146 = Delete(path (use dialog)=w359, entire hierarchy (F)=TRUE, error in=w356) -> (deleted path=w358:path, error out=w357:errorcluster)  [unwired: 2 in, 1 out]
          }
        }
        n147 = Build Array (concatenate)(w329, w315) -> (w322:string[])
        n148 = Concatenate Strings("HTML Help Source\\" ("string"), w329, ".htm" ("string")) -> (w333:string)
        n149 = Create Folder(path (use dialog)=w323, error in=w338) -> (created path=w325:path, error out=w324:errorcluster)  [unwired: 1 in, 1 out]
        n150 = call "Call HTML Help Generation Functions Async.vi"("error in (no error)"=w324, "Extra Page Names"=w322, "Destination Base Path"=w325) -> ("error out"=w321:errorcluster, "Destination Base Path Out (dup)"=w320:path)  [unwired: 7 in]
        n151 = Build Path(base path=w325, name or relative path="Build CHM.cfg") -> (appended path=w335:path)
        n152 = call <vilib>:"Open Config Data.vi"("error in (no error)"=w321, "configuration file path"=w335) -> ("error out"=w350:errorcluster, "refnum"=w349:T13)  [unwired: 7 in, 1 out]
        n153 = call-poly <vilib>:"Write Key.vi"("section"=w344, "error in (no error)"=w350, "value"=w318, "key"="Title", "refnum"=w349) -> ("error out"=w347:errorcluster, "refnum out"=w346:T13)  [unwired: 4 in, 1 out]
        n154 = call-poly <vilib>:"Write Key.vi"("section"=w344, "error in (no error)"=w347, "value"=w333, "key"="Default Topic", "refnum"=w346) -> ("error out"=w343:errorcluster, "refnum out"=w341:T13)  [unwired: 4 in, 1 out]
        n155 = call-poly <vilib>:"Write Key.vi"("section"=w344, "error in (no error)"=w343, "value"=w320, "key"="Base Path", "refnum"=w341) -> ("error out"=w342:errorcluster, "refnum out"=w340:T13)  [unwired: 4 in, 1 out]
        n156 = call <vilib>:"Close Config Data.vi"("error in (no error)"=w342, "refnum"=w340) -> ("error out"=w330:errorcluster)  [unwired: 8 in, 1 out]
      }
      frame "Project - Read project file content" {
        w372 = -1  # Read all lines
        w371 = T12."open"  # operation
        w370 = enum16{"read/write", "read-only", "write-only"}."read-only"  # access
        # "Open the project file and read the complete content."
        n157 = call-poly "Constants Main.vi"("Action"=Common."ProjectTemplatePathAndName") -> ("Output"=w363:string)  [unwired: 10 in]
        n158 = String To Path(string=w363) -> (path=w364:path)
        n159 = Open/Create/Replace File(file path (use dialog)=w364, error in=w361, operation (0:open)=w371, access (0:read/write)=w370) -> (refnum out=w368:refnum<file>, error out=w369:errorcluster)  [unwired: 3 out]
        n160 = Read from Text File(file (use dialog)=w368, count=w372, error in=w369) -> (refnum out=w362:refnum<file>, text=w366:string[], error out=w367:errorcluster)  [unwired: 2 out]
        n161 = Close File(refnum=w362) -> ()  [unwired: 1 in, 2 out]
      }
      frame "Project - Edit Utility section" {
        # "Edit the entries for the utility folder. Also added CHM pre build action entries"
        n162 = call-poly "Constants Main.vi"("Action"=Utility_folder."Utility.FolderName") -> ("Output"=w379:string)  [unwired: 10 in]
        n163 = call-poly "Constants Main.vi"("Action"=Utility_folder."Utility.Copy .llb to NI VeriStand dir.FileName") -> ("Output"=w380:string)  [unwired: 10 in]
        n164 = call-poly "Constants Main.vi"("Action"=Utility_folder."Utility.LLB Pre Build.FilePathAndName") -> ("Output"=w377:string)  [unwired: 10 in]
        n165 = String To Path(string=w377) -> (path=w376:path)
        n166 = Strip Path(path=w376) -> (name=w375:string)  [unwired: 1 out]
        n167 = for "For Iterate over each line and change the placeholders for the Utility entries." {
          tunnel: w385 -> [w397] mode=indexing
          shift-right: [w393] -> w383
          shift-left: w374 -> [w395]
          tunnel: [w391] -> w384 mode=indexing
          tunnel: w380 -> [w396]
          tunnel: w379 -> [w394]
          tunnel: w375 -> [w387]
          w389 = TRUE  # ignore case?
          w390 = TRUE  # replace all?
          w400 = "%CopyLLBtoNIVSFileName%"  # search
          w402 = "%UtilityFolderName%"  # search
          # "CHM Build VI as pre-build action"
          # "Copy .LLB to NI VeriStand dir.vi"
          # "Utility"
          n168 = Search and Replace String(replace all?=w390, case sensitive?=w389, input string=w397, search string=w402, replace string=w394, error in=w395) -> (result string=w401:string, error out=w399:errorcluster)  [unwired: 2 in, 2 out]
          n169 = Search and Replace String(replace all?=w390, case sensitive?=w389, input string=w401, search string=w400, replace string=w396, error in=w399) -> (result string=w392:string, error out=w398:errorcluster)  [unwired: 2 in, 2 out]
          n170 = Search and Replace String(replace all?=w390, case sensitive?=w389, input string=w392, search string="%CHMPreBuild%" ("result string"), replace string=w387, error in=w398) -> (result string=w391:string, error out=w393:errorcluster)  [unwired: 2 in, 2 out]
        }
      }
      frame "Project - Edit XML section" {
        # "Edit the Name and Path for the XML file."
        n171 = property class="Consolidated_CD"(reference=w405) -> ("Project Name"=w404:string, "Accessors:CD Template"=w403:refnum<class "NIVS_CD Template.lvclass">)  [unwired: 1 in, 2 out]
        n172 = call "XML - Get XML file name.vi"("CD Template"=w403, "CD Name"=w404) -> ("XML file name"=w407:string)  [unwired: 9 in]
        n173 = for "Iterate over each line and change the placeholder for the XML file name." {
          tunnel: w410 -> [w418] mode=indexing
          shift-right: [w417] -> w411
          shift-left: w406 -> [w413]
          tunnel: [w416] -> w409 mode=indexing
          tunnel: w407 -> [w412]
          w414 = TRUE  # ignore case?
          w415 = TRUE  # replace all?
          w419 = "%XMLCustomDeviceFileName%"  # search
          n174 = Search and Replace String(replace all?=w415, case sensitive?=w414, input string=w418, search string=w419, replace string=w412, error in=w413) -> (result string=w416:string, error out=w417:errorcluster)  [unwired: 2 in, 2 out]
        }
      }
      frame "Project - Edit Engine Library section" {
        # "Edit the entries for the Engine Library (Library name and folder name)"
        n175 = property class="Consolidated_CD"(reference=w421) -> ("Project Name"=w420:string)  [unwired: 1 in, 2 out]
        n176 = call "Change Engine Library Placeholders in project.vi"("error in (no error)"=w425, "Project Name"=w420, "Project file content in"=w422) -> ("error out"=w424:errorcluster, "Project file content out"=w426:string[])  [unwired: 7 in]
      }
      frame "Project - Edit Shared Library section" {
        # "Edit the entries for the Shared Library (Library name and folder name)"
        n177 = property class="Consolidated_CD"(reference=w428) -> ("Project Name"=w427:string)  [unwired: 1 in, 2 out]
        n178 = call-poly "Constants Main.vi"("Action"=CD_Shared_lvlib."LibraryFileName") -> ("Output"=w436:string)  [unwired: 10 in]
        n179 = call-poly "Constants Main.vi"("Action"=CD_Shared_lvlib."LibraryFolderName") -> ("Output"=w432:string)  [unwired: 10 in]
        n180 = call-poly "Constants Main.vi"("Action"=CD_Shared_lvlib."Shared.FolderName") -> ("Output"=w431:string)  [unwired: 10 in]
        n181 = Format Into String(format string=w436, w427) -> (resulting string=w433:string)  [unwired: 2 in, 1 out]
        n182 = for "Iterate over each line and change the placeholder for the Shared Library file and folder name." {
          tunnel: w434 -> [w455] mode=indexing
          shift-right: [w448] -> w439
          shift-left: w429 -> [w454]
          tunnel: [w449] -> w440 mode=indexing
          tunnel: w433 -> [w443]
          tunnel: w432 -> [w442]
          tunnel: w431 -> [w441]
          w446 = "%SharedLibrarySubfolderName%"  # search
          w452 = "%SharedLibraryFolderName%"  # search
          w444 = TRUE  # ignore case?
          w445 = TRUE  # replace all?
          w456 = "%SharedLibraryFileName%"  # search
          # "Shared"
          # "Shared"
          # "<CD> Shared.lvlib"
          n183 = Search and Replace String(replace all?=w445, case sensitive?=w444, input string=w455, search string=w456, replace string=w443, error in=w454) -> (result string=w453:string, error out=w451:errorcluster)  [unwired: 2 in, 2 out]
          n184 = Search and Replace String(replace all?=w445, case sensitive?=w444, input string=w453, search string=w452, replace string=w442, error in=w451) -> (result string=w450:string, error out=w447:errorcluster)  [unwired: 2 in, 2 out]
          n185 = Search and Replace String(replace all?=w445, case sensitive?=w444, input string=w450, search string=w446, replace string=w441, error in=w447) -> (result string=w449:string, error out=w448:errorcluster)  [unwired: 2 in, 2 out]
        }
      }
      frame "Project - Edit System Explorer Library section" {
        # "Edit the entries for the System Explorer Library (Library name and folder name)"
        n186 = property class="Consolidated_CD"(reference=w458) -> ("Project Name"=w457:string)  [unwired: 1 in, 2 out]
        n187 = call-poly "Constants Main.vi"("Action"=CD_System_Explorer_lvlib."LibraryFileName") -> ("Output"=w465:string)  [unwired: 10 in]
        n188 = Format Into String(format string=w465, w457) -> (resulting string=w468:string)  [unwired: 2 in, 1 out]
        n189 = call-poly "Constants Main.vi"("Action"=CD_System_Explorer_lvlib."System Explorer.FolderName") -> ("Output"=w470:string)  [unwired: 10 in]
        n190 = call-poly "Constants Main.vi"("Action"=CD_System_Explorer_lvlib."LibraryFolderName") -> ("Output"=w469:string)  [unwired: 10 in]
        n191 = for "Iterate over each line and change the placeholder for the System Explorer Library file and folder name." {
          tunnel: w461 -> [w485] mode=indexing
          shift-right: [w477] -> w463
          shift-left: w459 -> [w484]
          tunnel: [w478] -> w462 mode=indexing
          tunnel: w468 -> [w473]
          tunnel: w469 -> [w472]
          tunnel: w470 -> [w471]
          w474 = "%SystemExplorerSubfolderName%"  # search
          w482 = "%SystemExplorerLibraryFolderName%"  # search
          w476 = TRUE  # ignore case?
          w475 = TRUE  # replace all?
          w486 = "%SystemExplorerLibraryFileName%"  # search
          n192 = Search and Replace String(replace all?=w475, case sensitive?=w476, input string=w485, search string=w486, replace string=w473, error in=w484) -> (result string=w483:string, error out=w481:errorcluster)  [unwired: 2 in, 2 out]
          n193 = Search and Replace String(replace all?=w475, case sensitive?=w476, input string=w483, search string=w482, replace string=w472, error in=w481) -> (result string=w479:string, error out=w480:errorcluster)  [unwired: 2 in, 2 out]
          n194 = Search and Replace String(replace all?=w475, case sensitive?=w476, input string=w479, search string=w474, replace string=w471, error in=w480) -> (result string=w478:string, error out=w477:errorcluster)  [unwired: 2 in, 2 out]
        }
      }
      frame "Project - Edit Custom Device Name" {
        # "Edit the Custom Device name"
        n195 = property class="Consolidated_CD"(reference=w488) -> ("Project Name"=w487:string)  [unwired: 1 in, 2 out]
        n196 = for "Iterate over each line and change the placeholder for the Custom Device name." {
          tunnel: w490 -> [w500] mode=indexing
          shift-right: [w495] -> w492
          shift-left: w493 -> [w496]
          tunnel: [w499] -> w491 mode=indexing
          tunnel: w487 -> [w494]
          w497 = TRUE  # ignore case?
          w498 = TRUE  # replace all?
          w501 = "%CustomDeviceName%"  # search
          # "<CD>"
          n197 = Search and Replace String(replace all?=w498, case sensitive?=w497, input string=w500, search string=w501, replace string=w494, error in=w496) -> (result string=w499:string, error out=w495:errorcluster)  [unwired: 2 in, 2 out]
        }
      }
      frame "Project - Edit System Explorer LLB Name" {
        # "Edit the name for the System Explorer LLB."
        n198 = property class="Consolidated_CD"(reference=w503) -> ("Project Name"=w502:string)  [unwired: 1 in, 2 out]
        n199 = call-poly "Constants Main.vi"("Action"=Build_Spec_System_Explorer."Destinations.LLBFileName") -> ("Output"=w510:string)  [unwired: 10 in]
        n200 = Format Into String(format string=w510, w502) -> (resulting string=w507:string)  [unwired: 2 in, 1 out]
        n201 = for "Iterate over each line and change the placeholder for the System Explorer LLB." {
          tunnel: w507 -> [w517]
          tunnel: w506 -> [w515] mode=indexing
          tunnel: [w514] -> w505 mode=indexing
          shift-right: [w513] -> w511
          shift-left: w504 -> [w516]
          w512 = "%SystemExplorerLLBFileName%"  # search
          w518 = TRUE  # ignore case?
          w519 = TRUE  # replace all?
          # "<CD> Configuration.llb"
          n202 = Search and Replace String(replace all?=w519, case sensitive?=w518, input string=w515, search string=w512, replace string=w517, error in=w516) -> (result string=w514:string, error out=w513:errorcluster)  [unwired: 1 in, 3 out]
        }
      }
      frame "Project - Edit Engine LLB OS dependent file name" {
        n203 = property class="Consolidated_CD"(reference=w521) -> ("Project Name"=w520:string)  [unwired: 1 in, 2 out]
        n204 = call-poly "Constants Main.vi"("Action"=Build_Spec_Engine."Destinations.LLBLinux64FileName") -> ("Output"=w531:string)  [unwired: 10 in]
        n205 = call-poly "Constants Main.vi"("Action"=Build_Spec_Engine."Destinations.LLBLinuxARMFileName") -> ("Output"=w532:string)  [unwired: 10 in]
        n206 = call-poly "Constants Main.vi"("Action"=Build_Spec_Engine."Destinations.LLBPharlapFileName") -> ("Output"=w537:string)  [unwired: 10 in]
        n207 = call-poly "Constants Main.vi"("Action"=Build_Spec_Engine."Destinations.LLBWindowsFileName") -> ("Output"=w542:string)  [unwired: 10 in]
        n208 = call-poly "Constants Main.vi"("Action"=Build_Spec_Engine."Destinations.LLBVxWorksFileName") -> ("Output"=w538:string)  [unwired: 10 in]
        n209 = Format Into String(format string=w531, w520) -> (resulting string=w525:string)  [unwired: 2 in, 1 out]
        n210 = Format Into String(format string=w532, w520) -> (resulting string=w526:string)  [unwired: 2 in, 1 out]
        n211 = Format Into String(format string=w542, w520) -> (resulting string=w529:string)  [unwired: 2 in, 1 out]
        n212 = Format Into String(format string=w538, w520) -> (resulting string=w528:string)  [unwired: 2 in, 1 out]
        n213 = Format Into String(format string=w537, w520) -> (resulting string=w527:string)  [unwired: 2 in, 1 out]
        n214 = Build Array(w529, w528, w527, w526, w525) -> (w524:string[])
        n215 = for {
          shift-right: [w547] -> w534
          shift-left: w522 -> [w548]
          tunnel: w535 -> [w544] mode=indexing
          tunnel: w524 -> [w545]
          tunnel: [w543] -> w523 mode=indexing
          n216 = for {
            shift-right: [w556] -> w547
            shift-left: w548 -> [w555]
            shift-right: [w552] -> w543
            shift-left: w544 -> [w551]
            tunnel: string[] ["%EngineLLBWindowsFileName%", "%EngineLLBVxWorksFileName%", "%EngineLLBPharlapFileName%", "%EngineLLBLinuxARMFileName%", "%EngineLLBLinux64FileName%"] -> [w550] mode=indexing
            tunnel: w545 -> [w549] mode=indexing
            w553 = TRUE  # ignore case?
            w554 = TRUE  # replace all?
            n217 = Search and Replace String(replace all?=w554, case sensitive?=w553, input string=w551, search string=w550, replace string=w549, error in=w555) -> (result string=w552:string, error out=w556:errorcluster)  [unwired: 1 in, 3 out]
          }
        }
      }
      frame "Project - Write new project file" {
        # "Create new file and write the project file content into it."
        n218 = property class="Consolidated_CD"(reference=w559) -> ("Project Name"=w558:string, "Project Root"=w557:path)  [unwired: 1 in, 2 out]
        n219 = call-poly "Constants Main.vi"("Action"=Common."ProjectName") -> ("Output"=w583:string)  [unwired: 10 in]
        n220 = Format Into String(format string=w583, w558) -> (resulting string=w594:string)  [unwired: 2 in, 1 out]
        n221 = Build Path(base path=w557, name or relative path=w594) -> (appended path=w589:path)
        n222 = Open/Create/Replace File(file path (use dialog)=w589, error in=w560, operation (0:open)=T12."replace or create") -> (refnum out=w591:refnum<file>, error out=w590:errorcluster)  [unwired: 3 in, 1 out]
        n223 = Write to Text File(file (use dialog)=w591, text=w586, error in=w590) -> (refnum out=w588:refnum<file>, error out=w587:errorcluster)  [unwired: 2 out]
        n224 = Close File(refnum=w588, error in=w587) -> (path=w584:path, error out=w582:errorcluster)
        n225 = invoke class="App" method="Project.Open"(error in=w582, "Path"=w584) -> (error out=w577:errorcluster, "Project:Open"=w576:refnum<vi>)  [unwired: 2 in, 2 out]
        n226 = Build Path(base path=w557, name or relative path=path "Help") -> (appended path=w570:path)
        n227 = property class="Project"(reference=w576, error in=w577) -> (reference out=w575:refnum<vi>, error out=w573:errorcluster, "My Computer"=w574:refnum<vi>)
        n228 = invoke class="TargetItem" method="AddItem"(reference=w574, error in=w573, "Name"="Placeholder", "Path"=path "", "Type"="Folder") -> (reference out=w563:refnum<vi>, error out=w580:errorcluster, "AddItem"=w579:refnum<vi>)  [unwired: 1 in, 3 out]
        n229 = invoke class="ProjectItem" method="Convert to Auto-populating Folder"(reference=w579, error in=w580, "Path"=w570) -> (reference out=w565:refnum<vi>, error out=w561:errorcluster)  [unwired: 1 in, 2 out]
        n230 = Close Reference(reference=w565) -> (error out=w564:errorcluster)  [unwired: 1 in]
        n231 = invoke class="Project" method="Open Window"(reference=w575, error in=w561) -> (reference out=w562:refnum<vi>, error out=w566:errorcluster)  [unwired: 1 in, 1 out]
        n232 = Close Reference(reference=w563, error in (no error)=w564) -> ()  [unwired: 1 out]
        n233 = invoke class="Project" method="Save"(reference=w562, error in=w566) -> (reference out=w568:refnum<vi>, error out=w569:errorcluster)  [unwired: 2 in, 2 out]
        n234 = Close Reference(reference=w568, error in (no error)=w569) -> (error out=w567:errorcluster)
      }
    }
  }
  "error out" <- w6
